vi "Write VISA Instrument.vi"(8 "error in (no error)":errorcluster, 10 "VISA Instrument":refnum<visa-resource-name>, 11 "TektronixDPO_PhysicalDevice in":refnum<class "TektronixDPO_PhysicalDevice.lvclass">) -> (0 "error out":errorcluster, 3 "TektronixDPO_PhysicalDevice out":refnum<class "TektronixDPO_PhysicalDevice.lvclass">)   [LabVIEW 2013, in "TektronixDPO_PhysicalDevice.lvclass"]
uses:
  TektronixDPO_PhysicalDevice.lvclass
  TektronixDPO_PhysicalDevice.lvclass/TektronixDPO_PhysicalDevice.ctl
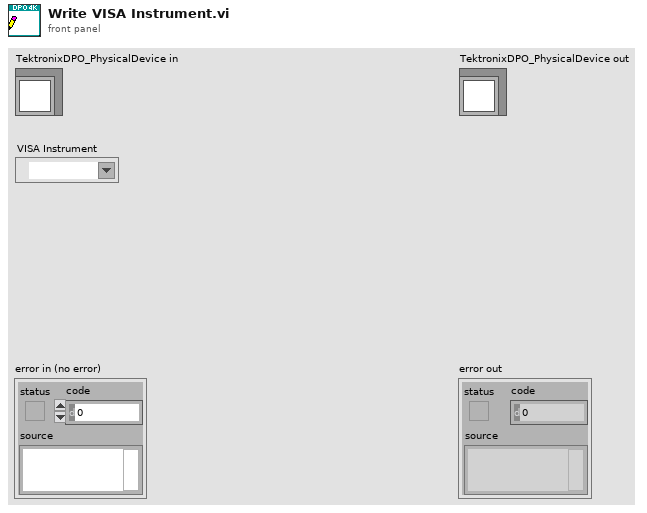
[diagram p1: front panel]
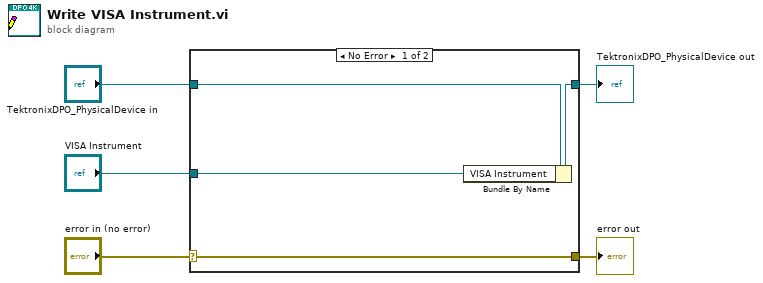
[diagram p0: block diagram]
diagram:
  n1 = case shown="No Error" "error in (no error)" {
    selector: "error in (no error)" -> [w9 w10]
    tunnel: [w9 w10] -> w4
    tunnel: [w7 w11] -> w2
    tunnel: "TektronixDPO_PhysicalDevice in" -> [w8 w11]
    tunnel: "VISA Instrument" -> [w6 _]
    frame No Error {
      n2 = Bundle By Name(cluster=w8, "VISA Instrument"=w6) -> (w7:refnum<class "TektronixDPO_PhysicalDevice.lvclass">)
    }
    frame Error {
    }
  }
  "error out" <- w4
  "TektronixDPO_PhysicalDevice out" <- w2
